vi "zdotu - Dot Product (CDB).vi"(5 "yInc":i32=1, 7 "xInc":i32=1, 10 "y":cdb[](array[numeric]), 11 "x":cdb[](array[numeric])) -> (0 "error":i32, 3 "zdotu":cdb)   [LabVIEW 2020, in "NI_AALBLAS.lvlib"]
doc: "Calculates the unconjugated dot product of two complex vectors."
uses:
  NI_AALBLAS.lvlib
  Fucntion.ctl
panel:
  # "zdotu=x'*y"
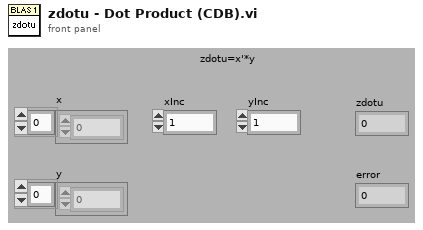
[diagram p1: front panel]
types:
  T1 = typedef "NI_AALBLAS.lvlib/fucntion.ctl" = u16
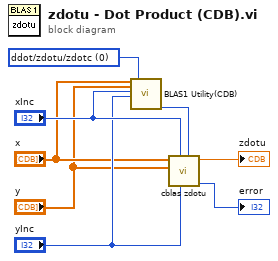
[diagram p0: block diagram]
diagram:
  w2 = T1 0 items=["ddot/zdotu/zdotc", "daxpy/zaxpy", "dnrm2/dznrm2", "dasum/dzasum", "dcopy/zcopy", "dswap/zswap", "drotm", "drot/zdrot", "idamax/izamax", "idamin/izamin", "dgemv/zgemv", "dsymv/zhemv", "dtrmv/ztrmv", "dsyr/zher", "dsyr2/zher2", "dger/zgeru/zgerc", "dtrsv/ztrsv", "dgemm/zgemm", "dsymm/zsymm/zhemm", "dtrmm/ztrmm", "dsyrk/zsyrk/zherk", "dsyr2k/zsyr2k/zher2k", "dtrsm/ztrsm"] ("function")
  n1 = call "BLAS1 Utility(CDB).vi"("x"="x", "y"="y", "xInc"="xInc", "yInc"="yInc", "function"=w2) -> ("n"=w1:i32)  [unwired: 14 in]
  n2 = call "cblas zdotu.vi"("n"=w1, "incy"="yInc", "incx"="xInc", "y"="y", "x"="x") -> ("error"=→"error":i32, "zdotu"=→"zdotu":cdb)  [unwired: 5 out]
